vi "WaitForResponse.vi"(6 "Timeout ms":i32, 8 "error in (no error)":errorcluster, 10 "Ack_Id":i32, 11 "NetworkConnection in":refnum<class "NetworkConnection.lvclass">) -> (0 "error out":errorcluster, 1 "ResponseReceived?":bool, 2 "StillConnected?":bool, 3 "NetworkConnection out":refnum<class "NetworkConnection.lvclass">, 4 "Timed Out?":bool)   [LabVIEW 2020, in "NetworkConnection.lvclass"]
doc: "Waits for the response from the remote system.\n\nJKI Network Streams Connection 1.1.1.15\nJavier Ruiz - JKI\nCopyright (c) 2020, JKI\n\nThis library is provided \"AS IS\" ,WITHOUT WARRANTIES OR CONDITIONS OF ANY KIND, either express or implied."
uses:
  NetworkConnection.lvclass
  NetworkConnection.lvclass/NetworkConnection.ctl
panel:
  # "Copyright © 2020 JKI All rights reserved.\n\nAuthor: Javier Ruiz <javier.ruiz@jki.net>\n\nThis library is provided \"AS IS\" ,WITHOUT WARRANTIES OR \nCONDITIONS OF ANY KIND, either expressed or implied.\n\nJKI -- jki.net"
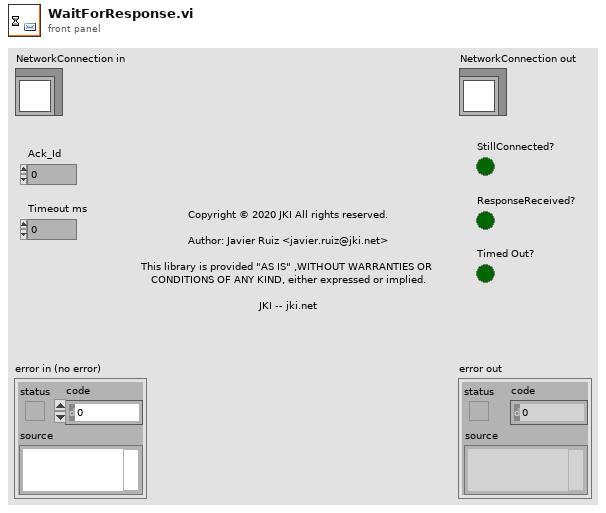
[diagram p1: front panel]
types:
  T1 = typedef "NetworkConnection.lvclass/NetworkMessage--Cluster.ctl" = cluster{"NetworkCommand":T2, "Wait for Ack?":bool, "Ack Id":i32}
  T2 = typedef "NetworkConnection.lvclass/NetworkCommand--Cluster.ctl" = cluster{"Command":string, "Arguments":variant, " Msg Id":i32}
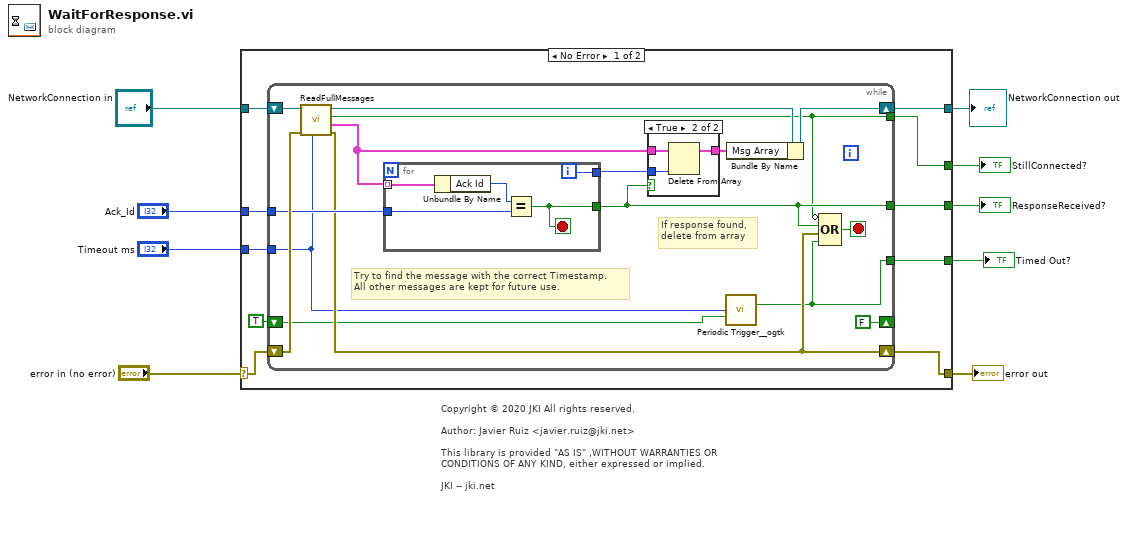
[diagram p0: block diagram]
diagram:
  # "Copyright © 2020 JKI All rights reserved.\n\nAuthor: Javier Ruiz <javier.ruiz@jki.net>\n\nThis library is provided \"AS IS\" ,WITHOUT WARRANTIES OR \nCONDITIONS OF ANY KIND, either expressed or implied.\n\nJKI -- jki.net"
  n1 = case shown="No Error" "error in (no error)" {
    selector: "error in (no error)" -> [w18 w46]
    tunnel: [w17 w46] -> w8
    tunnel: [w13 w45] -> w6
    tunnel: "NetworkConnection in" -> [w19 w45]
    tunnel: "Ack_Id" -> [w15 _]
    tunnel: "Timeout ms" -> [w16 _]
    tunnel: [w11 _] -> w3
    tunnel: [w14 _] -> w2
    tunnel: [w12 _] -> w1
    frame No Error {
      n2 = while {
        tunnel: w16 -> [w23]
        tunnel: w15 -> [w33]
        tunnel: [w20] -> w14
        tunnel: [w26] -> w12
        tunnel: [w27] -> w11
        shift-right: [w25] -> w17
        shift-left: w18 -> [w34]
        shift-right: [w31] -> w13
        shift-left: w19 -> [w35]
        shift-right: [FALSE] -> _
        shift-left: TRUE -> [w22]
        stop <- w24 stop-if-true
        # "If response found,\ndelete from array"
        # "Try to find the message with the correct Timestamp.\nAll other messages are kept for future use."
        n3 = call "ReadFullMessages.vi"("Timeout(ms)"=w23, "error in (no error)"=w34, "NetworkConnection in"=w35) -> ("error out"=w25:errorcluster, "Messages"=w30:T1[], "StillConnected?"=w26:bool, "NetworkConnection out"=w32:refnum<class "NetworkConnection.lvclass">)  [unwired: 4 in, 1 out]
        n4 = for {
          tunnel: w30 -> [w42] mode=indexing
          tunnel: w33 -> [w43]
          tunnel: [w41] -> w27
          tunnel: [w40] -> w29
          i -> [w40]
          stop <- w41 stop-if-true
          n5 = Unbundle By Name(w42) -> ("Ack Id"=w44:i32)
          n6 = Equal?(x=w44, y=w43) -> (x = y?=w41:bool)
        }
        n7 = case shown="True" w27 {
          tunnel: w30 -> [w36 w39]
          tunnel: w29 -> [_ w38]
          tunnel: [w36 w37] -> w28
          frame False {
          }
          frame True {
            n8 = Delete From Array(array=w39, index=w38) -> (array with subset deleted=w37:T1[])  [unwired: 1 in, 1 out]
          }
        }
        n9 = call "Periodic Trigger__ogtk.vi"("time (ms)"=w23, "reset"=w22) -> ("Triggered"=w20:bool)  [unwired: 11 in, 2 out]
        n10 = Bundle By Name(cluster=w32, "Msg Array"=w28) -> (w31:refnum<class "NetworkConnection.lvclass">)
        n11 = Compound Arithmetic op=OR(invert w26, w27, w25, w20) -> (w24:bool)
      }
    }
    frame Error {
    }
  }
  "error out" <- w8
  "NetworkConnection out" <- w6
  "ResponseReceived?" <- w3
  "Timed Out?" <- w2
  "StillConnected?" <- w1
